vi "LVH5Rdereference.vi"   [LabVIEW 2017]
doc: "Opens the HDF5 object referenced."
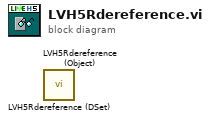
[diagram p0: block diagram]
diagram:
  n1 = call <vilib>:"LVH5Rdereference (DSet).vi"() -> ()  [unwired: 7 in, 3 out]
  n2 = call <vilib>:"LVH5Rdereference (Object).vi"() -> ()  [unwired: 7 in, 3 out]
